vi "cm2nm_initialize_new_session.vi"(0 "Sample locations of Interest":refnum<vi>, 1 "Sample_Information":T1, 2 "Session File":path, 3 "Instrument":u16, 4 "Session Name/ID":string, 5 "Notes_out":string) -> (6 "Sample_out":T1, 7 "Current Session Information":T2, 8 "Fiducial Count":u32[](array[numeric]))   [LabVIEW 2011]
doc: "Initialize the program for a new session including the spot vs. session table, fiducial count indicator, and the current and sample out fields."
uses:
  cm2nm_sample_set.ctl
  cm2nm_coordinate_information_v2.ctl
  Instrument_type_enum_v2.ctl
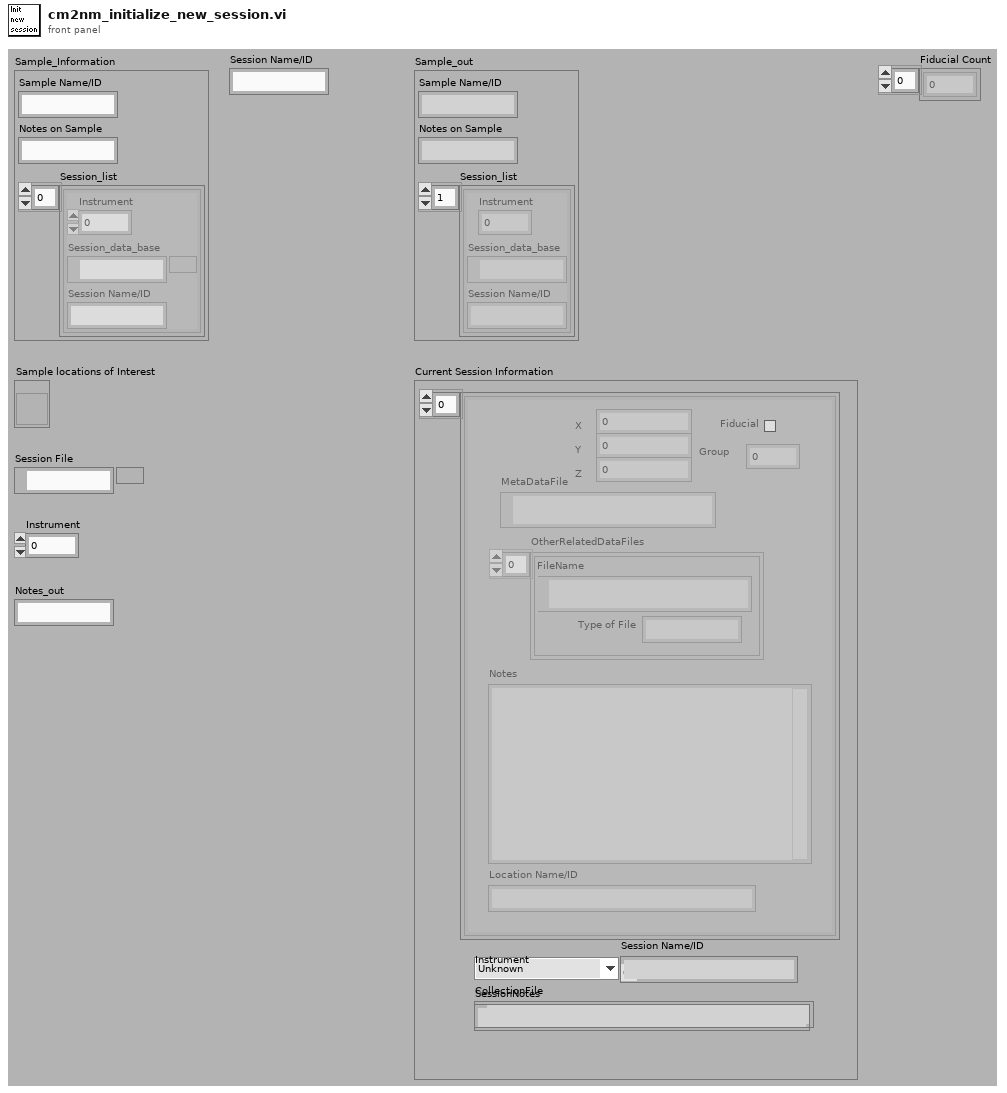
[diagram p1: front panel]
types:
  T1 = cluster{"Sample Name/ID":string, "Notes on Sample":string, "Session_list":cluster{"Instrument":u16, "Session_data_base":path, "Session Name/ID":string}[]}
  T2 = typedef "cm2nm_sample_set.ctl" = cluster{"CollectionOfPoints":T3[], "Instrument":T4, "CollectionFile":path, "Session Name/ID":string, "SessionNotes":string}
  T3 = typedef "cm2nm_coordinate_information_v2.ctl" = cluster{"MetaDataFile":path, "X":dbl, "Y":dbl, "Z":dbl, "Group":i32, "Rotation":dbl[unit], "Fiducial":bool, "Magnification":dbl, "Working_Distance":dbl, "Notes":string, "Location Name/ID":string, "OtherRelatedDataFiles":cluster{"Type of File":string, "FileName":path}[], "Available":bool}
  T4 = typedef "Instrument_type_enum_v2.ctl" = enum16{"Unknown", "Philips FEI SEM IRC", "JEOL 7000F EML_MFC", "MXRD MFC", "JEOL_EPMA"}
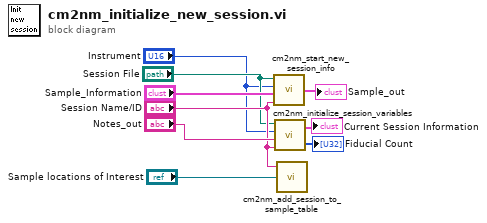
[diagram p0: block diagram]
diagram:
  n1 = call "cm2nm_start_new_session_info.vi"("Session Name/ID_out"="Session Name/ID", "Sample_Information"="Sample_Information", "Instrument_out"="Instrument", "Session File_out"="Session File") -> ("Sample_out"=→"Sample_out":T1)
  n2 = call "cm2nm_initialize_session_variables.vi"("Session Name/ID_out"="Session Name/ID", "Notes_out"="Notes_out", "Instrument_out"="Instrument", "Session File_out"="Session File") -> ("Fiducial Count"=→"Fiducial Count":u32[], "Current Session Information"=→"Current Session Information":T2)
  n3 = call "cm2nm_add_session_to_sample_table.vi"("Sample locations of Interest"="Sample locations of Interest", "Session Name/ID_out"="Session Name/ID") -> ()  [unwired: 2 out]
